vi "Duplicate.vi"(8 "error in":errorcluster, 10 "parameters":variant, 11 "Thermo Channel in":refnum<class "Thermo Channel.lvclass">) -> (0 "error out":errorcluster, 3 "Thermo Channel copy":refnum<class "Thermo Channel.lvclass">)   [LabVIEW 2025, in "Thermo.lvlib" / "Thermo Channel.lvclass"]
doc: "Implements the specific behavior of a node when it is being duplicated\nCan be used to change the name of the new node for example adding Copy to it. \nCopyright 2017 National Instruments Corporation\n\nLicensed under the Apache License, Version 2.0 (the \"License\"); you may not use this file except in compliance with the License. You may obtain a copy of the License at http://www.apache.org/licenses/LICENSE-2.0\nUnless required by applicable law or agreed to in writing, software distributed under the License is distributed on an \"AS IS\" BASIS, WITHOUT WARRANTIES OR CONDITIONS OF ANY KIND, either express or implied. See the License for the specific language governing permissions and limitations under the License."
uses:
  Thermo Channel.lvclass
  Thermo Channel.lvclass/Thermo Channel.ctl
  Thermo Channel configuration/Thermo Channel configuration.lvclass
  Users/Public/Documents/Sandia National Labs/TSS Plugin/Abstract Engine.lvlibp/Abstract Channel/Abstract Channel.lvclass
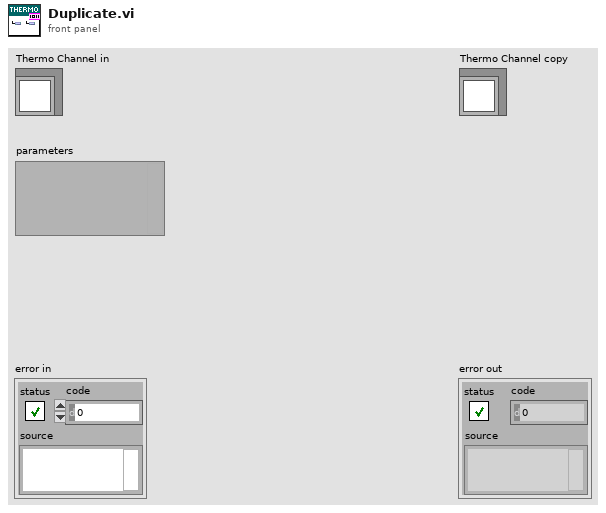
[diagram p1: front panel]
types:
  T1 = typedef "Abstract Engine.lvlibp/Channel configuration.lvclass/Default Channel.ctl" = cluster{"Address":string, "SW Alias":string, "Enabled":bool, "Type":string, "Description":string}
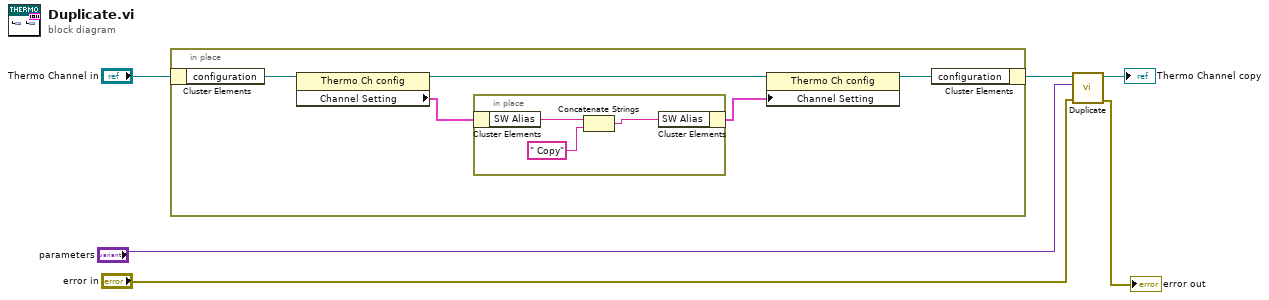
[diagram p0: block diagram]
diagram:
  n1 = in-place {
    n2 = in-place-cluster #1("Thermo Channel in") -> ("configuration"=w11:refnum<class "Thermo Channel configuration.lvclass">)
    n3 = property class="Thermo Ch config"(reference=w11) -> (reference out=w9:refnum<class "Thermo Channel configuration.lvclass">, "Channel Setting"=w8:T1)  [unwired: 1 in, 1 out]
    n4 = in-place {
      n5 = in-place-cluster #2(w8) -> ("SW Alias"=w13:string)
      n6 = Concatenate Strings(w13, " Copy") -> (w12:string)
      n7 = in-place-cluster #2("SW Alias"=w12) -> (w7:T1)
    }
    n8 = property class="Thermo Ch config"(reference=w9, "Channel Setting"=w7) -> (reference out=w10:refnum<class "Thermo Channel configuration.lvclass">)  [unwired: 1 in, 1 out]
    n9 = in-place-cluster #1("configuration"=w10) -> (w6:refnum<class "Thermo Channel.lvclass">)
  }
  n10 = call-parent "Duplicate.vi"("error in"="error in", "parameters"="parameters", "CEF_Serialize node in"=w6) -> ("error out"=→"error out":errorcluster, "CEF_Serialize node out"=→"Thermo Channel copy":refnum<class "Thermo Channel.lvclass">)  [unwired: 7 in]
